vi "Get Active Cell Position.vi"(6 "Active Cell In":T1 caption="活动单元格:活动单元格", 8 "错误输入":errorcluster, 11 "Mlistbox Ref":refnum<vi>) -> (0 "错误输出":errorcluster, 2 "CellPos Out":T2 caption="活动单元格:位置", 3 "Mlistbox Ref Dup":refnum<vi>)   [LabVIEW 2012, in "Mlistbox Tools.lvlib"]
uses:
  Mlistbox Tools.lvlib
  <vilib>/Utility/miscctls.llb/LVPositionTypeDef.ctl
  <vilib>/Utility/miscctls.llb/LVRowAndColumnTypeDef.ctl
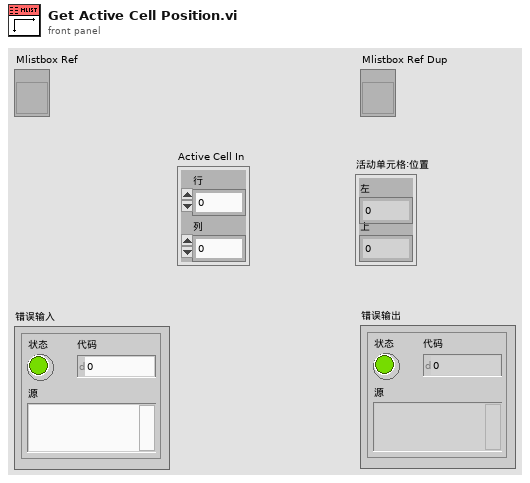
[diagram p1: front panel]
types:
  T1 = typedef "LVRowAndColumnTypeDef.ctl" = cluster{"Row":i32, "Column":i32}
  T2 = typedef "LVPositionTypeDef.ctl" = cluster{"Left":i32, "Top":i32}
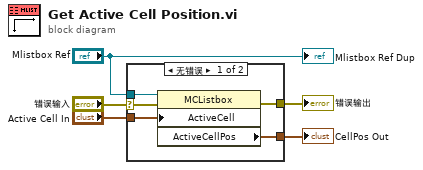
[diagram p0: block diagram]
diagram:
  n1 = case shown="无错误" "错误输入" {
    selector: "错误输入" -> [w9 w11]
    tunnel: [w8 w11] -> w4
    tunnel: "Mlistbox Ref" -> [w10 _]
    tunnel: [w7 _] -> w2
    tunnel: "Active Cell In" -> [w6 _]
    frame No Error {
      n2 = property class="MCListbox"(reference=w10, error in=w9, "ActiveCell"=w6) -> (error out=w8:errorcluster, "ActiveCellPos"=w7:T2)  [unwired: 1 out]
    }
    frame Error {
    }
  }
  "错误输出" <- w4
  "CellPos Out" <- w2
  "Mlistbox Ref Dup" <- "Mlistbox Ref"
